vi "initDigitalOutTasks.vi"(4 "Digital Out - Config File":path=path "C:/Users/DAQ/Desktop/Labview Joost/Jon Code/DigiOut.txt", 5 "General HardWare Constants":T2={"Nr. of Columns"=1, "Nr. of Rows"=18, "OverSampling"=10, "Fetch Rate "=20, "Sampling Rate"=0, "Nr. of BNC inputs"=3, "Sample Strip Length"=10}, 6 "Digital Out Tasks":tag[](array[tag])=["PXI1Slot2/port0/line0:7", "PXI1Slot3/port0/line0:7"], 7 "Reference Clock Properties":T3={"RefClockGlobalName"="/PXI1Slot2/PXI_Clk10", "RefClockRate"=100000.0}, 8 "Error In":errorcluster, 10 "Switch Bitorder?":bool, 11 "Counter Setup":T1={"Device and Counter"="PXI1Slot3/ctr0", "PXI_trigger"="PXI_Trig3"}) -> (0 "Error Out":errorcluster, 1 "BitMaskValues out":u32[][](array[numeric]), 2 "BitMask Out":bool[][][](array[boolean]), 3 "DigitalTasks OUT":refnum<k21>[](array[refnum]))   [LabVIEW 2011]
uses:
  controls/RefClockSettings.ctl
  controls/General Hardware config.ctl
  controls/Counter Setup.ctl
  <vilib>/DAQmx/write.llb/DAQmx Write (Digital 1D U32 1Chan NSamp).vi
  <vilib>/Utility/file.llb/Read From Spreadsheet File (I64).vi
  <vilib>/DAQmx/create/channels.llb/DAQmx Create Channel (CO-Pulse Generation-Ticks).vi
  <vilib>/DAQmx/configure/timing.llb/DAQmx Timing (Implicit).vi
  <vilib>/DAQmx/configure/events/hardwareSignals.llb/DAQmx Export Signal (Most Signals).vi
  <vilib>/DAQmx/create/channels.llb/DAQmx Create Channel (DO-Digital Output).vi
  <vilib>/DAQmx/configure/timing.llb/DAQmx Timing (Sample Clock).vi
  <vilib>/DAQmx/miscellaneous.llb/DAQmx Fill In Error Info.vi
  C:/Program Files/National Instruments/LabVIEW 2011/resource/objmgr/daqmx.rc
panel:
  # "Array"
  # "Acq. System"
  # "Other analog Input"
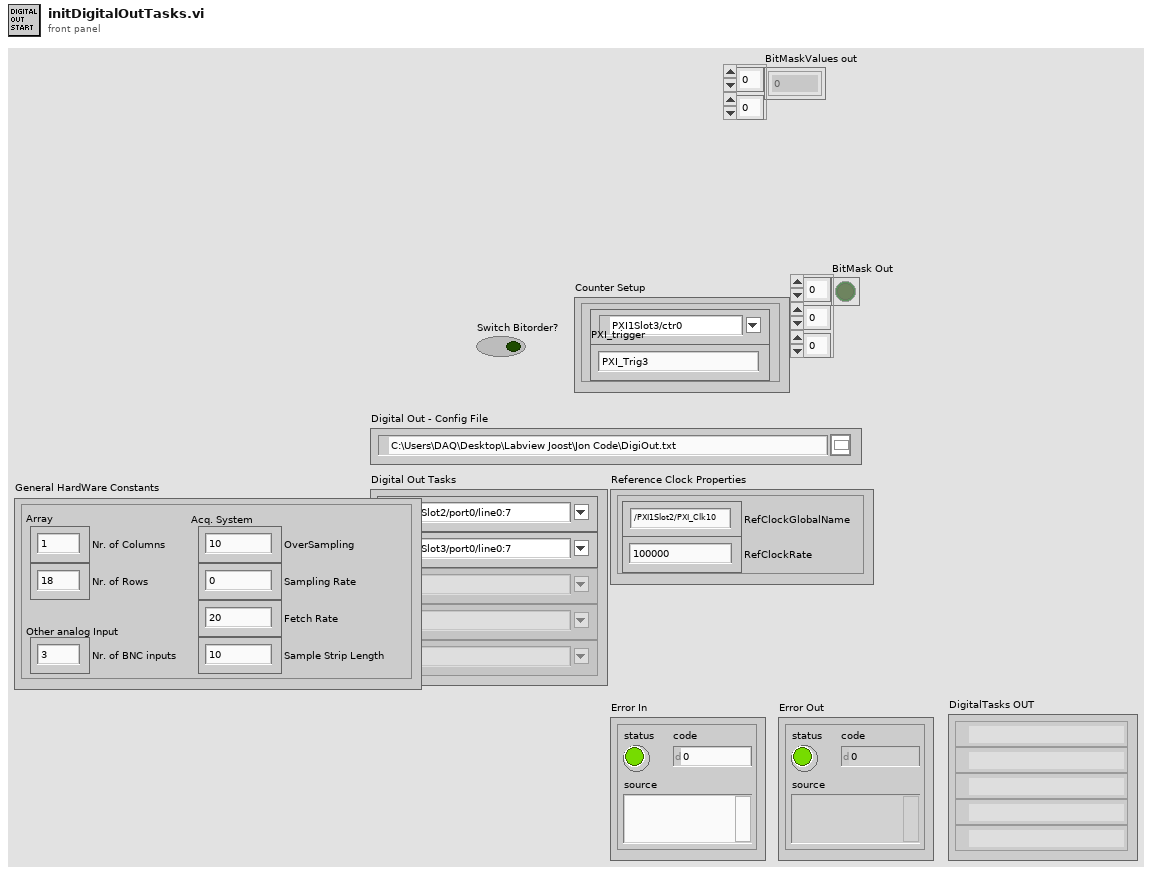
[diagram p1: front panel]
types:
  T1 = typedef "Counter Setup.ctl" = cluster{"Device and Counter":tag, "PXI_trigger":string}
  T2 = typedef "General Hardware config.ctl" = cluster{"Nr. of Columns":i32, "Nr. of Rows":i32, "OverSampling":i32, "Fetch Rate ":i32, "Sampling Rate":i32, "Nr. of BNC inputs":i32, "Sample Strip Length":i32}
  T3 = typedef "RefClockSettings.ctl" = cluster{"RefClockGlobalName":string, "RefClockRate":dbl}
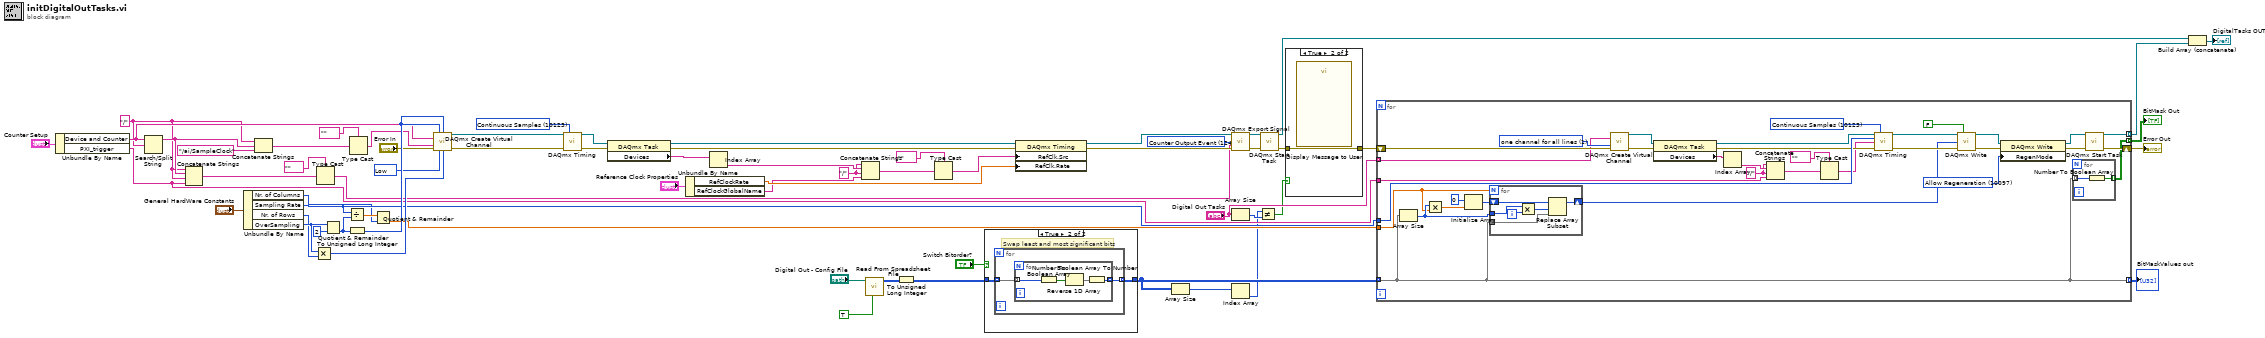
[diagram p0: block diagram]
diagram:
  w22 = "/" ("search string/char (-)")
  w33 = "/"
  w50 = 10214 items=["High"=10192, "Low"=10214] ("idle state")
  w60 = 12494 items=["AI Convert Clock"=12484, "10MHz Reference Clock"=12536, "20MHz Timebase Clock"=12486, "Sample Clock"=12487, "Advance Trigger"=12488, "Reference Trigger"=12490, "Start Trigger"=12491, "Advance Complete Event"=12492, "AI Hold Complete Event"=12493, "Counter Output Event"=12494, "Change Detection Event"=12511, "Watchdog Timer Expired Event"=12512] ("signal")
  w58 = 10123 items=["Finite Samples"=10178, "Continuous Samples"=10123] ("sample mode")
  n1 = Unbundle By Name("Counter Setup") -> ("Device and Counter"=w28:tag, "PXI_trigger"=w19:string)
  n2 = Search/Split String(string=w28, search string/char (-)=w22) -> (substring before match=w26:string)  [unwired: 1 in, 2 out]
  n3 = Concatenate Strings(w22, w26, w22, w19) -> (w25:string)
  n4 = Unbundle By Name("General HardWare Constants") -> ("Nr. of Columns"=w11:i32, "Sampling Rate"=w14:i32, "Nr. of Rows"=w35:i32, "OverSampling"=w36:i32)
  n5 = Concatenate Strings(w22, w26, "/ai/SampleClock") -> (w29:string)
  n6 = Multiply(x=w36, y=w35) -> (x*y=w34:i32)
  n7 = Type Cast(type=tag "", x=w25) -> (*(type *) &x=w23:tag)
  n8 = Quotient & Remainder(x=w36, y=2) -> (floor(x/y)=w13:i32)  [unwired: 1 out]
  n9 = Divide(x=w14, y=w13) -> (x/y=w12:dbl)
  n10 = To Unsigned Long Integer(number=w13) -> (unsigned 32bit integer=w53:u32)
  n11 = Type Cast(type=tag "", x=w29) -> (*(type *) &x=w27:tag)
  n12 = Quotient & Remainder(x=w12, y=w11) -> (floor(x/y)=w10:dbl)  [unwired: 1 out]
  n13 = call-poly <vilib>:"DAQmx Create Virtual Channel.vi"("high ticks"=w53, "low ticks"=w53, "counter"=w28, "source of ticks"=w27, "error in"="Error In", "idle state"=w50, "initial delay"=w34) -> ("task out"=w57:refnum<k21>, "error out"=w56:errorcluster)  [unwired: 7 in]
  n14 = call-poly <vilib>:"DAQmx Timing.vi"("task/channels in"=w57, "sample mode"=w58, "error in"=w56) -> ("task out"=w43:refnum<k21>, "error out"=w44:errorcluster)  [unwired: 11 in]
  n15 = property class="DAQmx Task"(reference=w43, error in=w44) -> (reference out=w42:refnum<k21>, error out=w41:errorcluster, "Devices"=w39:tag[])
  n16 = Unbundle By Name("Reference Clock Properties") -> ("RefClockRate"=w49:dbl, "RefClockGlobalName"=w32:string)
  n17 = Index Array(array=w39) -> (element=w46:tag)  [unwired: 1 in]
  n18 = Concatenate Strings(w33, w46, w33, w32) -> (w38:string)
  n19 = call-poly <vilib>:"Read From Spreadsheet File.vi"("transpose (no:F)"=TRUE, "file path (dialog if empty)"="Digital Out - Config File") -> ("all rows"=w21:i64[][])  [unwired: 5 in, 4 out]
  n20 = To Unsigned Long Integer(number=w21) -> (unsigned 32bit integer=w17:u32[][])
  n21 = Type Cast(type=tag "", x=w38) -> (*(type *) &x=w40:tag)
  n22 = case shown="True" "Switch Bitorder?" {
    tunnel: w17 -> [w66 w68]
    tunnel: [w66 w67] -> w8
    frame False {
    }
    frame True {
      # "Swap least and most significant bits"
      n23 = for {
        tunnel: w68 -> [w70] mode=indexing
        tunnel: [w69] -> w67 mode=indexing
        n24 = for {
          tunnel: w70 -> [w74] mode=indexing
          tunnel: [w71] -> w69 mode=indexing
          n25 = Number To Boolean Array(number=w74) -> (Boolean array=w73:bool[])
          n26 = Reverse 1D Array(array=w73) -> (reversed array=w72:bool[])
          n27 = Boolean Array To Number(Boolean array=w72) -> (number=w71:u32)
        }
      }
    }
  }
  n28 = property class="DAQmx Timing"(reference=w42, error in=w41, "RefClk.Src"=w40, "RefClk.Rate"=w49) -> (reference out=w48:refnum<k21>, error out=w47:errorcluster)
  n29 = Array Size(array=w8) -> (size(s)=w6:i32[])
  n30 = call-poly <vilib>:"DAQmx Export Signal.vi"("task/channels in"=w48, "signal"=w60, "output terminal"=w23, "error in"=w47) -> ("task out"=w59:refnum<k21>, "error out"=w51:errorcluster)  [unwired: 10 in]
  n31 = Array Size(array="Digital Out Tasks") -> (size(s)=w7:i32)
  n32 = Index Array(array=w6) -> (element=w3:i32)  [unwired: 1 in]
  n33 = Not Equal?(x=w3, y=w7) -> (x != y?=w4:bool)
  n34 = call <vilib>:"DAQmx Start Task.vi"("task/channels in"=w59, "error in"=w51) -> ("task out"=w55:refnum<k21>, "error out"=w5:errorcluster)  [unwired: 12 in]
  n35 = case shown="True" w4 {
    tunnel: w5 -> [w75 w76]
    tunnel: [w75 w76] -> w2
    frame False {
    }
    frame True {
      n36 = call "Display Message to User"() -> ()  [unwired: 10 in, 2 out]
    }
  }
  n37 = for {
    tunnel: w8 -> [w77] mode=indexing
    tunnel: w14 -> [w108]
    tunnel: "Digital Out Tasks" -> [w95] mode=indexing
    shift-right: [w110] -> w63
    shift-left: w2 -> [w109]
    tunnel: [w94] -> w62 mode=indexing
    tunnel: [w82] -> w18 mode=indexing
    tunnel: w19 -> [w79]
    tunnel: w10 -> [w78]
    tunnel: [w77] -> w1 mode=indexing
    w80 = "/"
    w100 = 10097 items=["Allow Regeneration"=10097, "Do Not Allow Regeneration"=10158] ("RegenMode")
    w105 = 1 items=["one channel for each line", "one channel for all lines"] ("line grouping")
    w107 = 10123 items=["Finite Samples"=10178, "Continuous Samples"=10123, "Hardware Timed Single Point"=12522] ("sample mode")
    n38 = Array Size(array=w77) -> (size(s)=w96:i32)
    n39 = Multiply(x=w96, y=w78) -> (x*y=w98:dbl)
    n40 = Initialize Array(u32 0, w98) -> (w97:u32[])
    n41 = for {
      N: w78 -> [_]
      shift-right: [w117] -> w81
      shift-left: w97 -> [w118]
      tunnel: w77 -> [w113]
      tunnel: w96 -> [w115]
      i -> [w116]
      n42 = Multiply(x=w115, y=w116) -> (x*y=w114:i32)
      n43 = Replace Array Subset(array=w118, new element=w113, index=w114) -> (w117:u32[])
    }
    n44 = call-poly <vilib>:"DAQmx Create Virtual Channel.vi"("lines"=w95, "line grouping"=w105, "error in"=w109) -> ("task out"=w87:refnum<k21>, "error out"=w86:errorcluster)  [unwired: 11 in]
    n45 = property class="DAQmx Task"(reference=w87, error in=w86) -> (reference out=w84:refnum<k21>, error out=w85:errorcluster, "Devices"=w90:tag[])
    n46 = Index Array(array=w90) -> (element=w88:tag)  [unwired: 1 in]
    n47 = Concatenate Strings(w80, w88, w80, w79) -> (w91:string)
    n48 = Type Cast(type=tag "", x=w91) -> (*(type *) &x=w83:tag)
    n49 = call-poly <vilib>:"DAQmx Timing.vi"("task/channels in"=w84, "sample mode"=w107, "rate"=w108, "source"=w83, "error in"=w85) -> ("task out"=w106:refnum<k21>, "error out"=w104:errorcluster)  [unwired: 9 in]
    n50 = call-poly <vilib>:"DAQmx Write.vi"("task/channels in"=w106, "auto start"=FALSE, "data"=w81, "error in"=w104) -> ("task out"=w102:refnum<k21>, "error out"=w93:errorcluster)  [unwired: 9 in, 1 out]
    n51 = property class="DAQmx Write"(reference=w102, error in=w93, "RegenMode"=w100) -> (reference out=w101:refnum<k21>, error out=w92:errorcluster)
    n52 = for {
      tunnel: [w111] -> w82 mode=indexing
      tunnel: w77 -> [w112] mode=indexing
      n53 = Number To Boolean Array(number=w112) -> (Boolean array=w111:bool[])
    }
    n54 = call <vilib>:"DAQmx Start Task.vi"("task/channels in"=w101, "error in"=w92) -> ("task out"=w94:refnum<k21>, "error out"=w110:errorcluster)  [unwired: 12 in]
  }
  "Error Out" <- w63
  "BitMask Out" <- w18
  "BitMaskValues out" <- w1
  n55 = Build Array (concatenate)(w55, w62) -> (→"DigitalTasks OUT":refnum<k21>[])
